vi "Send Burner Status.vi"(5 "Main Timer":dbl, 8 "error in (no error)":errorcluster, 11 "Timer Application Data":T1) -> (0 "error out":errorcluster, 3 "Timer Application Data Output":T1)   [LabVIEW 2023]
uses:
  controls/Burner Duty Cycle.ctl
  controls/Timer Application Cluster.ctl
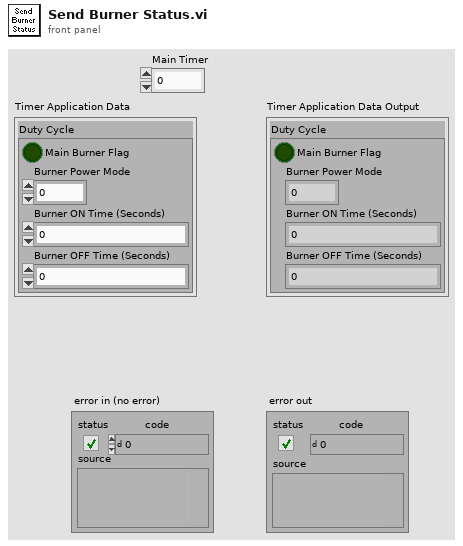
[diagram p1: front panel]
types:
  T1 = typedef "Timer Application Cluster.ctl" = cluster{"Duty Cycle":T2}
  T2 = typedef "Burner Duty Cycle.ctl" = cluster{"Burner ON Time (Seconds)":dbl, "Burner OFF Time (Seconds)":dbl, "Main Burner Flag":bool, "Burner Power Mode":u8}
  T3 = typedef "Timers.ctl" = cluster{"Main Timer":dbl, "Burner Status":bool}
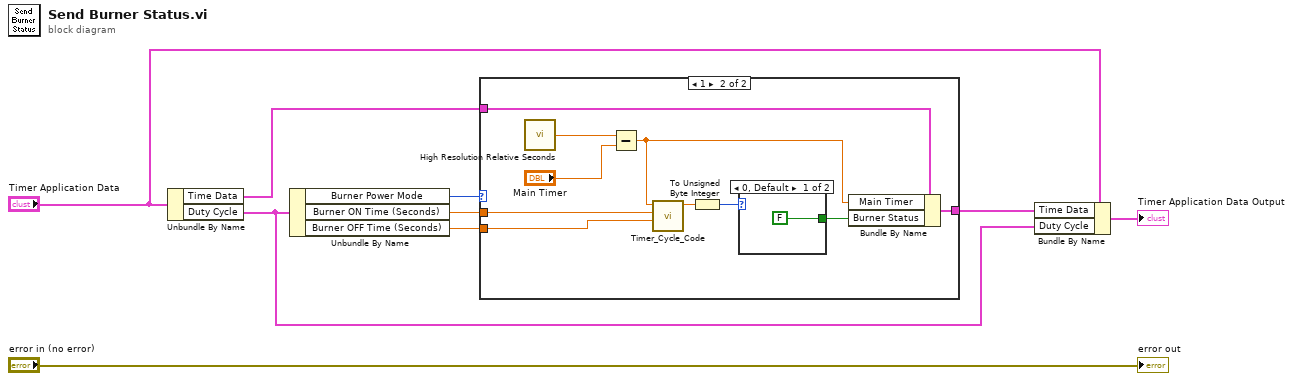
[diagram p0: block diagram]
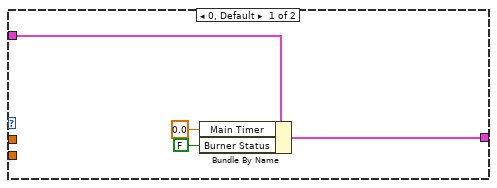
[diagram p2: hidden frame]
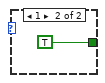
[diagram p3: hidden frame]
diagram:
  n1 = Unbundle By Name("Timer Application Data") -> ("Time Data"=w5:T3, "Duty Cycle"=w1:T2)
  n2 = Unbundle By Name(w1) -> ("Burner Power Mode"=w6:u8, "Burner ON Time (Seconds)"=w8:dbl, "Burner OFF Time (Seconds)"=w7:dbl)
  n3 = case shown="1" w6 {
    tunnel: [w12 w23] -> w3
    tunnel: w5 -> [w13 w22]
    tunnel: w8 -> [_ w19]
    tunnel: w7 -> [_ w18]
    frame 0, Default {
      n4 = Bundle By Name(cluster=w13, "Main Timer"=0.0, "Burner Status"=FALSE) -> (w12:T3)
    }
    frame 1 {
      n5 = call <vilib>:"High Resolution Relative Seconds.vi"() -> ("relative seconds"=w20:dbl)
      n6 = Subtract(x=w20, y="Main Timer") -> (x-y=w14:dbl)
      n7 = call "Timer_Cycle_Code.vi"("Burner OFF Time (Seconds)"=w18, "Burner ON Time (Seconds)"=w19, "Timer"=w14) -> ("burner_state"=w17:dbl)  [unwired: 8 in]
      n8 = To Unsigned Byte Integer(number=w17) -> (unsigned 8bit integer=w16:u8)
      n9 = case shown="0, Default" w16 {
        tunnel: [FALSE TRUE] -> w15
        frame 0, Default {
        }
        frame 1 {
        }
      }
      n10 = Bundle By Name(cluster=w22, "Main Timer"=w14, "Burner Status"=w15) -> (w23:T3)
    }
  }
  n11 = Bundle By Name(cluster="Timer Application Data", "Time Data"=w3, "Duty Cycle"=w1) -> (→"Timer Application Data Output":T1)
  "error out" <- "error in (no error)"
